vi "plc read write.vi"(7 "CMd To PLC":string, 8 "error In":errorcluster, 11 "connection ID IN":refnum<k5>) -> (0 "error out":errorcluster, 2 "Data Out":string, 3 "connection ID OUT":refnum<k5>)   [LabVIEW 2015]
panel:
  out "bytes written1":i32
  # "ee"
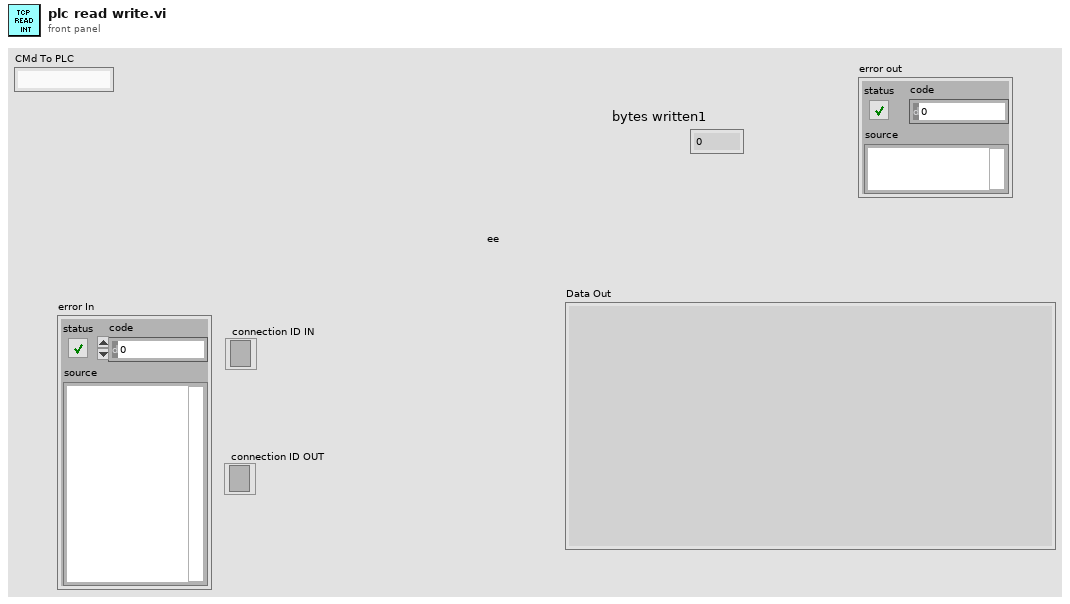
[diagram p1: front panel]
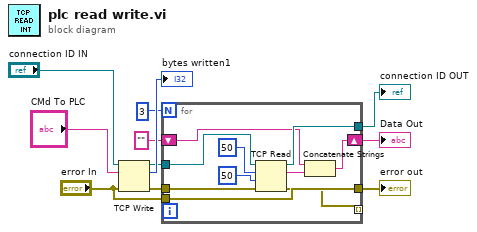
[diagram p0: block diagram]
diagram:
  n1 = TCP Write(connection ID="connection ID IN", data in="CMd To PLC", error in (no error)="error In") -> (connection ID out=w5:refnum<k5>, bytes written=→"bytes written1":i32, error out=w4:errorcluster)  [unwired: 1 in]
  n2 = for {
    N: 3 -> [_]
    tunnel: w5 -> [w21]
    tunnel: w4 -> [w20]
    tunnel: [w19] -> w2
    tunnel: [w13] -> w3
    shift-right: [w14] -> w6
    shift-left: "" ("data out") -> [w16]
    tunnel: "error In" -> [w13]
    tunnel: [w12] -> _ mode=indexing
    n3 = TCP Read(connection ID=w21, bytes to read=50, error in (no error)=w20, 9:50 ("timeout ms (25000)")) -> (connection ID out=w19:refnum<k5>, data out=w15:string, error out=w12:errorcluster)  [unwired: 1 in]
    n4 = Concatenate Strings(w16, w15) -> (w14:string)
  }
  "Data Out" <- w6
  "error out" <- w3
  "connection ID OUT" <- w2
